vi "Upload Logo_General_UI.vi"(8 "error in (no error)":errorcluster, 10 "logo path file":path=path "C:/Users/shanks75/Desktop/GTRON/Images/fcilogo(84x76).png", 11 "Picture in":refnum<vi>) -> (0 "error out":errorcluster)   [LabVIEW 2019, in "ZenGage v3.0 UI.lvclass"]
uses:
  ZenGage v3.0 UI.lvclass
  <vilib>/Utility/miscctls.llb/LVBoundsTypeDef.ctl
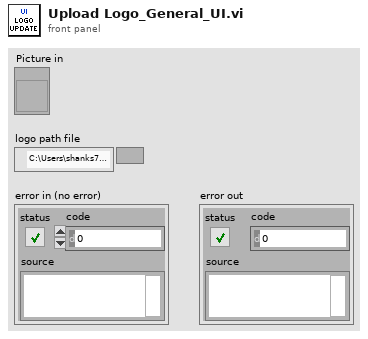
[diagram p1: front panel]
types:
  T1 = typedef "LVBoundsTypeDef.ctl" = cluster{"Width":u32, "Height":u32}
  T2 = typedef "imagedata.ctl" = cluster{"image type":i32, "image depth":i32, "image":u8[], "mask":u8[], "colors":u32[], "Rectangle":cluster{"left":i16, "top":i16, "right":i16, "bottom":i16}}
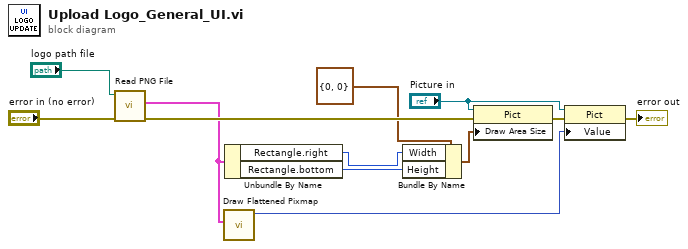
[diagram p0: block diagram]
diagram:
  n1 = call <vilib>:"Read PNG File.vi"("error in (no error)"="error in (no error)", "path to PNG file"="logo path file") -> ("error out"=w8:errorcluster, "image data"=w5:T2)  [unwired: 7 in, 1 out]
  n2 = call <vilib>:"Draw Flattened Pixmap.vi"("image data"=w5) -> ("new picture"=w10:picture)  [unwired: 8 in]
  n3 = Unbundle By Name(w5) -> ("Rectangle.right"=w2:i16, "Rectangle.bottom"=w3:i16)
  n4 = Bundle By Name(cluster=T1 {"Width"=0, "Height"=0} ("Draw Area Size"), "Width"=w2, "Height"=w3) -> (w1:T1)
  n5 = property class="Pict"(reference="Picture in", error in=w8, "Draw Area Size"=w1) -> (error out=w7:errorcluster)  [unwired: 1 out]
  n6 = property class="Pict"(reference="Picture in", error in=w7, "Value"=w10) -> (error out=→"error out":errorcluster)  [unwired: 1 out]
